vi "(SubVI)_Control_Save_Dpp_bin_MultiSite.vi"(6 "Vessel Number":dbl, 8 "Frm Indx":dbl, 9 "Frm#":dbl=1310.0, 10 "Dpp_bsln":dbl=1.5694465244142645e-05, 11 "refnum in":refnum<file>) -> (0 "error out":errorcluster, 3 "refnum out":refnum<file>)   [LabVIEW 2012]
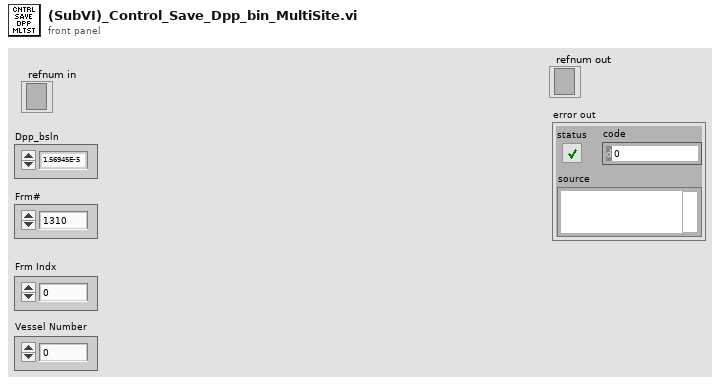
[diagram p1: front panel]
types:
  T1 = enum16{"big-endian, network order", "native, host order", "little-endian"}
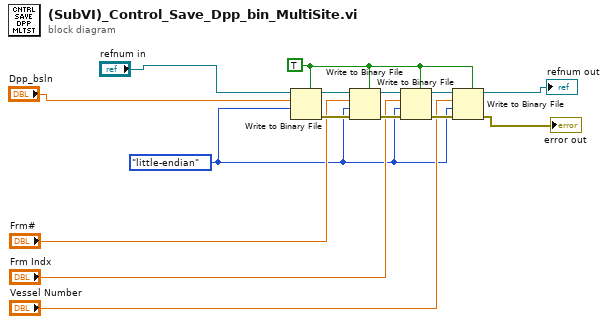
[diagram p0: block diagram]
diagram:
  w1 = T1."little-endian" ("byte order (0:big-endian, network order)")
  w2 = TRUE ("prepend array or string size? (T)")
  n1 = Write to Binary File(file (use dialog)="refnum in", data="Dpp_bsln", 5:w2, 9:w1) -> (refnum out=w15:refnum<file>, error out=w14:errorcluster)  [unwired: 2 in, 1 out]
  n2 = Write to Binary File(file (use dialog)=w15, data="Frm#", error in=w14, 5:w2, 9:w1) -> (refnum out=w9:refnum<file>, error out=w10:errorcluster)  [unwired: 1 in, 1 out]
  n3 = Write to Binary File(file (use dialog)=w9, data="Frm Indx", error in=w10, 5:w2, 9:w1) -> (refnum out=w7:refnum<file>, error out=w8:errorcluster)  [unwired: 1 in, 1 out]
  n4 = Write to Binary File(file (use dialog)=w7, data="Vessel Number", error in=w8, 5:w2, 9:w1) -> (refnum out=→"refnum out":refnum<file>, error out=→"error out":errorcluster)  [unwired: 1 in, 1 out]
